vi "PE7260_set_sensitivity.vi"(0 "Address":string, 1 "delay time":dbl, 2 "mode":dbl, 3 "SEN 7265":dbl) -> ()   [LabVIEW 2019]
panel:
  in  "read GPIB (false=on)":bool=TRUE
  out "7265":string="1.298E-05\r\n"
  # "1    2 nV \n2    5 nV\n3    10 nV\n4    20 nV\n5    50 nV\n6    100 nV \n7    200 nV\n8    500 nV\n9    1 muV\n10  2muV\n11  5 muV\n12  10 muV\n13  20 muV\n14  50 muV\n15  100 muV\n16  200 muV\n17  500 muV\n18  1 mV\n19  2 mV\n20  5mV\n21  10 mV\n22  20 mV\n23  50 mV\n24  100 mV\n25  200 mV\n26  500 mV\n27  1V"
  # "L\nI\n\n7\n2\n6\n5"
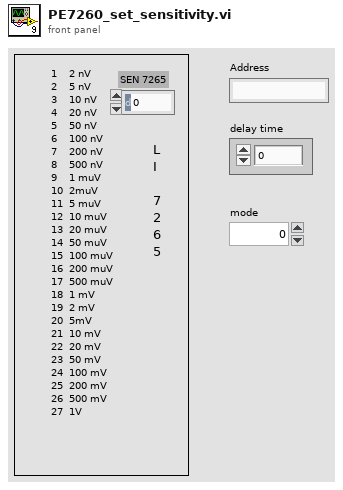
[diagram p1: front panel]
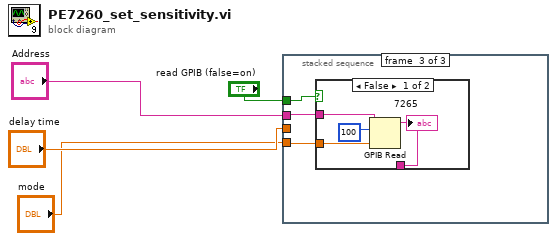
[diagram p0: block diagram]
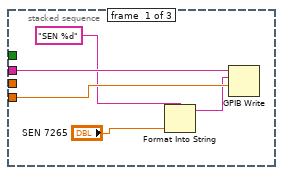
[diagram p2: hidden frame]
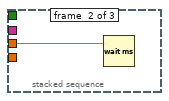
[diagram p3: hidden frame]
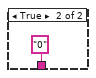
[diagram p4: hidden frame]
diagram:
  n1 = stacked-sequence {
    tunnel: "Address" -> [w9 _ w12]
    tunnel: "mode" -> [w8 _ w13]
    tunnel: "delay time" -> [_ w10 _]
    tunnel: "read GPIB (false=on)" -> [_ _ w11]
    frame #0 {
      n2 = Format Into String "Format Into String"(format string="SEN %d", "SEN 7265") -> (resulting string=w5:string)  [unwired: 2 in, 1 out]
      n3 = GPIB Write(0:w9, 1:w5, 2:w8) -> ()  [unwired: 2 in, 2 out]
    }
    frame #1 {
      n4 = Wait (ms)(milliseconds to wait=w10) -> ()  [unwired: 1 out]
    }
    frame #2 {
      n5 = case shown="False" w11 {
        tunnel: w13 -> [w16 _]
        tunnel: w12 -> [w15 _]
        tunnel: [w14 "0" ("data")] -> _
        frame False {
          n6 = GPIB Read(0:w15, 1:100, 2:w16) -> (5:w14:string)  [unwired: 2 in, 2 out]
          "7265" <- w14
        }
        frame True {
        }
      }
    }
  }
